vi "RVC 3-link serial robot Cylindrical.vi"() -> ()   [LabVIEW 2014]
uses:
  <vilib>/Analysis/Matrix/Datatypes/RealMatrix.ctl
  <vilib>/robotics/Kinematics/Analytical/Initialize Generic Serial Arm.vi
  <vilib>/robotics/Kinematics/Analytical/NI_Robotics_AnalyticKinematics.lvlib
  <vilib>/robotics/Kinematics/Robot/NI_Robotics_Serial Robot Arm.lvclass
  <vilib>/Analysis/Matrix/NI_Matrix.lvlib
panel:
  in  "appended array":dbl[](array[numeric])=[0.0, 0.0, 0.0]
  out "transformation":picture
  out "forward kinematics":T1
  out "3D Picture":refnum<vi>(3d-picture)
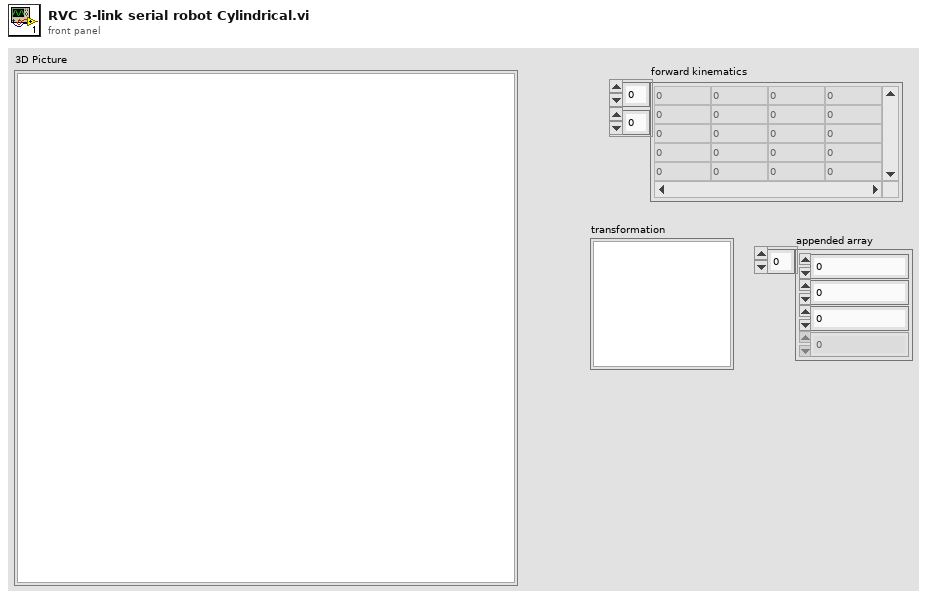
[diagram p1: front panel]
types:
  T1 = typedef "NI_Matrix.lvlib/RealMatrix.ctl" = dbl[][]
  T2 = typedef "DH Kinematic Parameters.ctl" = cluster{"twist angle":dbl, "length":dbl, "rotation angle":dbl, "offset distance":dbl, "joint type":T3, "joint coordinate offset":dbl}
  T3 = typedef "NI_Robotics_Link.lvclass/Joint Type.ctl" = enum16{"Revolute", "Prismatic"}
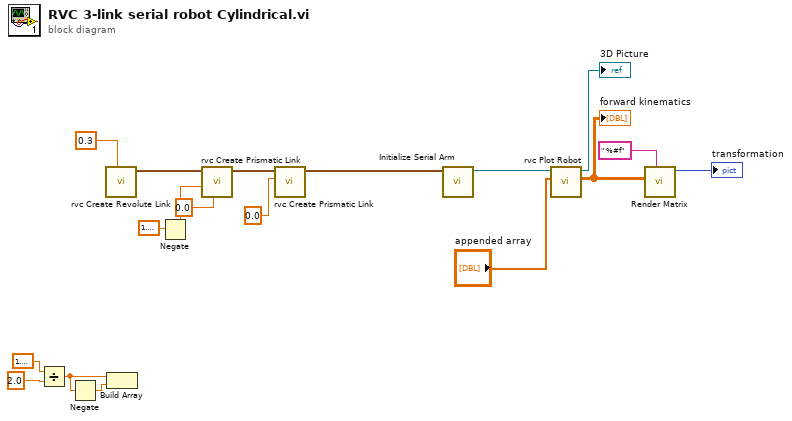
[diagram p0: block diagram]
diagram:
  n1 = Divide(x=1.5707963267948966, y=2.0) -> (x/y=w14:dbl)
  n2 = Negate(x=w14) -> (-x=w13:dbl)
  n3 = call "rvc Create Revolute Link.vi"("offset distance (d)"=0.3) -> ("Array"=w7:T2[])  [unwired: 10 in]
  n4 = Build Array(w14, w13) -> ()  [unwired: 1 out]
  n5 = Negate(x=1.5707963267948966) -> (-x=w1:dbl)
  n6 = call "rvc Create Prismatic Link.vi"("offset distance (d)"=0.0, "twist angle (alpha)"=w1, "Array 2"=w7) -> ("Array"=w8:T2[])  [unwired: 8 in]
  n7 = call "rvc Create Prismatic Link.vi"("length (a)"=0.0 ("offset distance (d)"), "Array 2"=w8) -> ("Array"=w6:T2[])  [unwired: 9 in]
  n8 = call-poly <vilib>:"Initialize Serial Arm.vi"("kinematic parameters"=w6) -> ("serial arm out"=w18:refnum<class "NI_Robotics_Serial Robot Arm.lvclass">)  [unwired: 9 in, 1 out]
  n9 = call "rvc Plot Robot.vi"("joint positions"="appended array", "NI_Robotics_Serial Robot Arm in"=w18) -> ("forward kinematics"=w10:T1, "Scene Object Out"=→"3D Picture":refnum<vi>)  [unwired: 7 in, 1 out]
  "forward kinematics" <- w10
  n10 = call "Render Matrix.vi"("format string"=" %#f", "A"=w10) -> ("picture out"=→"transformation":picture)  [unwired: 9 in]
